vi "Write Resource Name.vi"(8 "error in (no error)":errorcluster, 10 "Resource Name":refnum<k15>, 11 "IVI Oscilloscope in":refnum<class "IVI Oscilloscope.lvclass">) -> (0 "error out":errorcluster, 3 "IVI Oscilloscope out":refnum<class "IVI Oscilloscope.lvclass">)   [LabVIEW 2014, in "IVI Oscilloscope.lvclass"]
uses:
  IVI Oscilloscope.lvclass
  IVI Oscilloscope.lvclass/IVI Oscilloscope.ctl
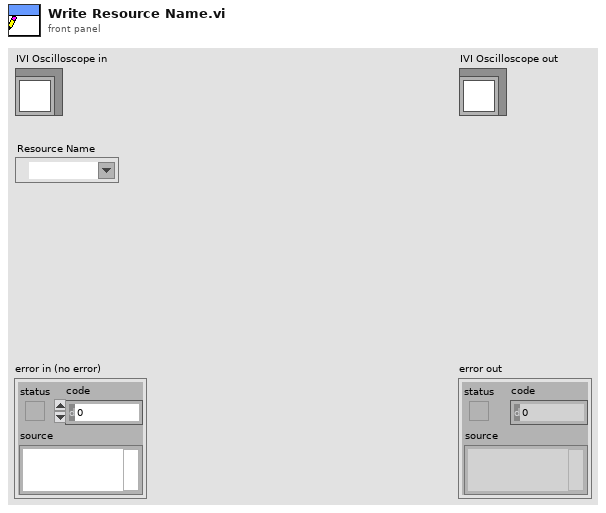
[diagram p1: front panel]
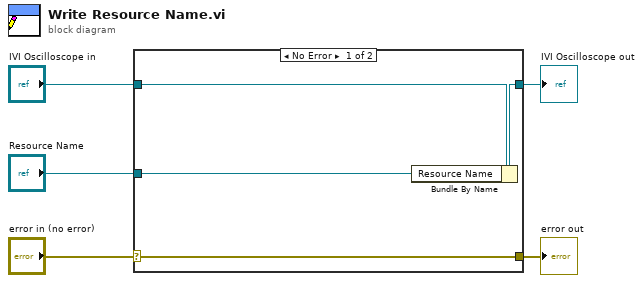
[diagram p0: block diagram]
diagram:
  n1 = case shown="No Error" "error in (no error)" {
    selector: "error in (no error)" -> [w9 w10]
    tunnel: [w9 w10] -> w4
    tunnel: [w7 w11] -> w2
    tunnel: "IVI Oscilloscope in" -> [w8 w11]
    tunnel: "Resource Name" -> [w6 _]
    frame No Error {
      n2 = Bundle By Name(cluster=w8, "Resource Name"=w6) -> (w7:refnum<class "IVI Oscilloscope.lvclass">)
    }
    frame Error {
    }
  }
  "error out" <- w4
  "IVI Oscilloscope out" <- w2
